vi "Read Config JSON.vi"(8 "error in (no error)":errorcluster, 10 "JSON Config":string, 11 "Abs_Type in":refnum<class "Abs_Type.lvclass">) -> (0 "error out":errorcluster, 3 "Abs_Type out":refnum<class "Abs_Type.lvclass">)   [LabVIEW 2021, in "Abs_Type.lvclass"]
uses:
  Abs_Type.lvclass
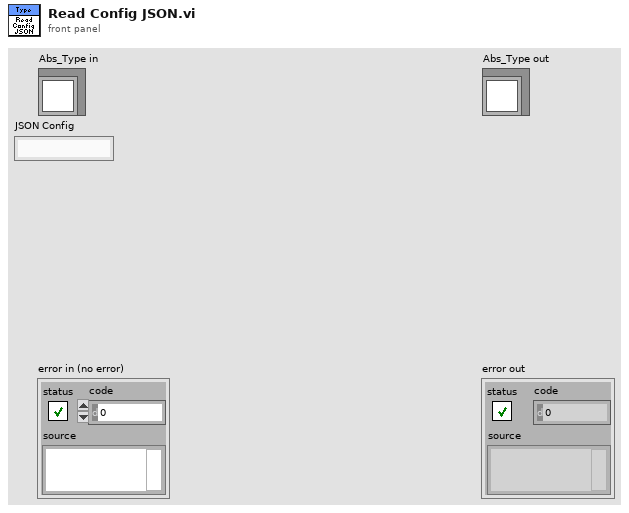
[diagram p1: front panel]
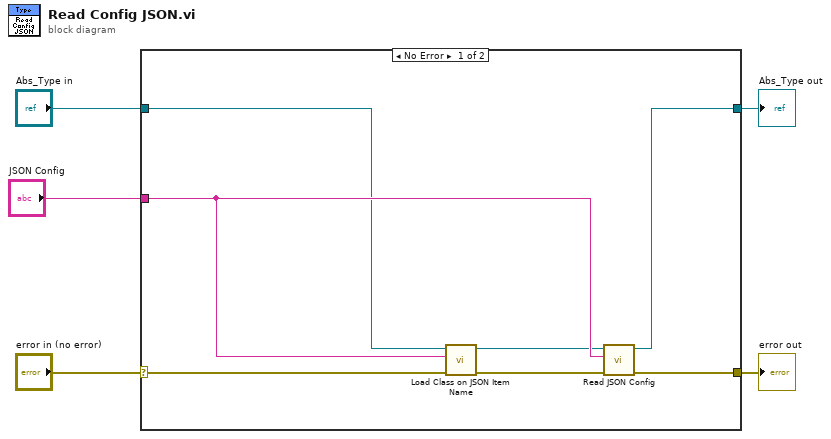
[diagram p0: block diagram]
diagram:
  n1 = case shown="No Error" "error in (no error)" {
    selector: "error in (no error)" -> [w10 w14]
    tunnel: [w11 w14] -> w4
    tunnel: [w12 w13] -> w2
    tunnel: "Abs_Type in" -> [w8 w13]
    tunnel: "JSON Config" -> [w9 _]
    frame No Error {
      n2 = call "Load Class on JSON Item Name.vi"("error in (no error)"=w10, "JSON Config"=w9, "Abs_Type in"=w8) -> ("error out"=w7:errorcluster, "Abs_Type out"=w6:refnum<class "Abs_Type.lvclass">)  [unwired: 7 in]
      n3 = call-dynamic "Read JSON Config.vi"("error in (no error)"=w7, "JSON Config"=w9, "Abs_Type in"=w6) -> ("error out"=w11:errorcluster, "Abs_Type out"=w12:refnum<class "Abs_Type.lvclass">)  [unwired: 7 in]
    }
    frame Error {
    }
  }
  "error out" <- w4
  "Abs_Type out" <- w2
